vi "Test_Multiple_SubPanel_Single HSMO_External_Control.vi"() -> ()   [LabVIEW 2021]
uses:
  C:/Program Files (x86)/Hyper State Machine Framework/SSW_Hyper_State_Machine.lvlibp/State_Machine_Class/Main_State_Machine/Hyper_State_Machine.lvclass
  Commander/Commander.lvclass
  Image_Acquisition/Image_Acquisition.lvclass
  Motion_Control/Motion_Control.lvclass
  DIO/DIO.lvclass
  Data_Logging/Data_Logging.lvclass
  Common_State/Common_State.lvclass
  C:/Program Files (x86)/Hyper State Machine Framework/SSW_Hyper_State_Machine.lvlibp/State_Machine_Class/State_Machine_Module.llb/State Machine.ctl
  C:/Program Files (x86)/Hyper State Machine Framework/SSW_Hyper_State_Machine.lvlibp/State_Machine_Class/State_Machine_Module.llb/Lock_Unlock.ctl
  C:/Program Files (x86)/Hyper State Machine Framework/SSW_Hyper_State_Machine.lvlibp
panel:
  out "VI_Path[]":path[](array[path])
  in  "Panel List":i32(listbox)
  in  "Change SubPanel":bool
  out "HSMO[]":refnum<class "Hyper_State_Machine.lvclass">[](array[class])
  out "Lock Status":enum32{"Unlock", "Lock"}[](array[radio])
  in  "Lock State":bool
  in  "Change Mode":bool=TRUE
  in  "Panel Index":i32
  in  "Show Stop Button":bool
  in  "UnLoad_Panel":bool
  in  "Load_Panel":bool
  in  "Time Target (s)":dbl=30.0 format="%#_13g"
  in  "System_Delay(s)":dbl=0.01 format="%.0p"
  in  "State_Interval_Time(s)":dbl format="%.0p"
  in  "Stop":bool=TRUE
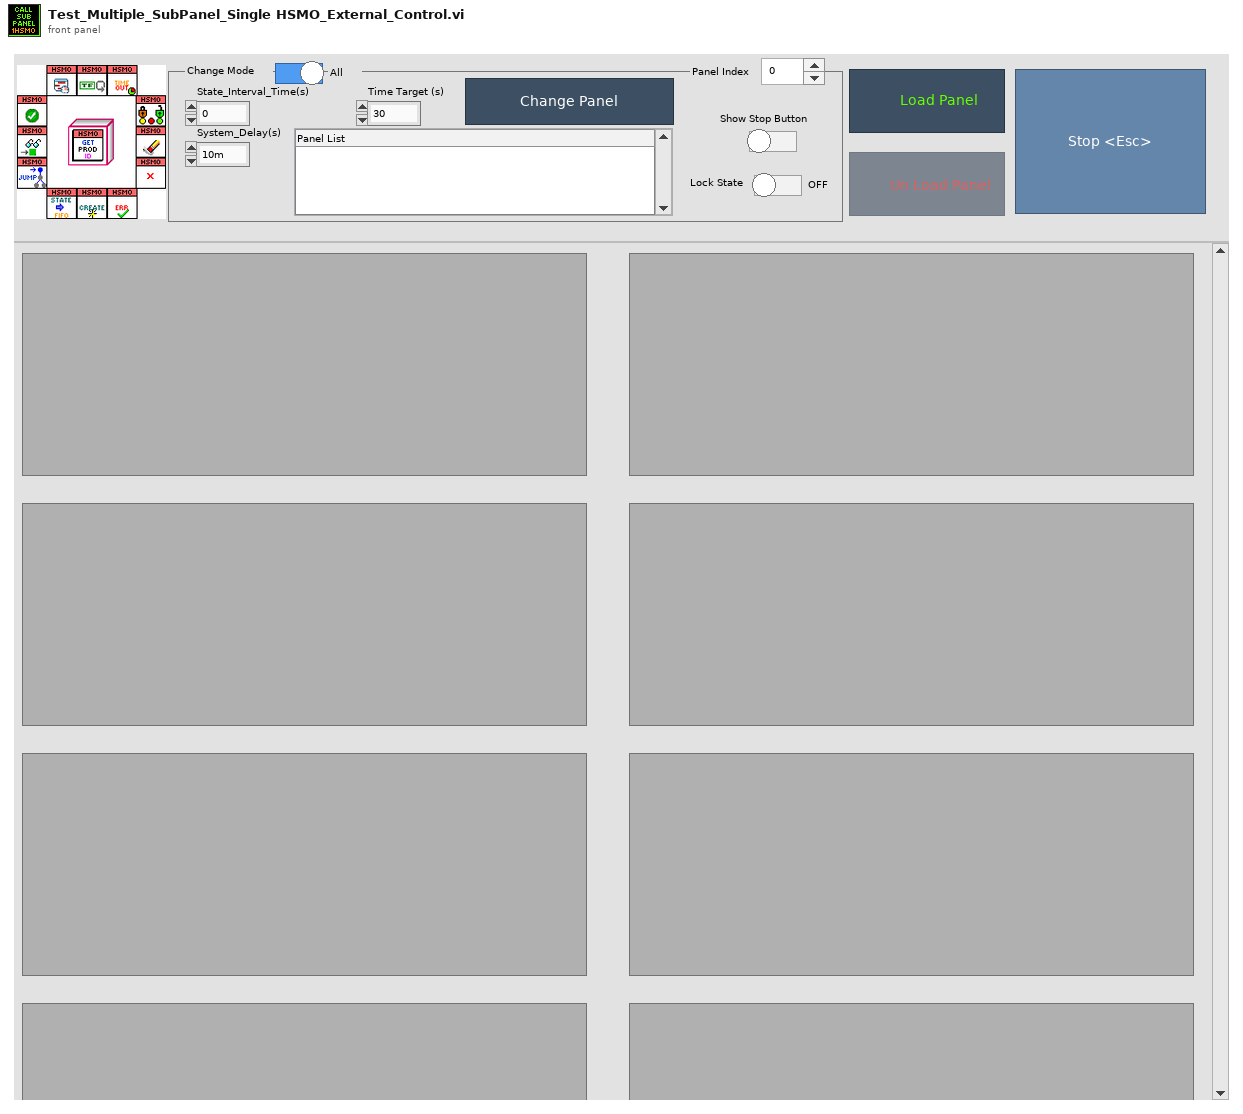
[diagram p1: front panel]
types:
  T1 = enum8{"Enabled", "Disabled", "Disabled and Grayed Out"}
  T2 = typedef "SSW_Hyper_State_Machine.lvlibp/State Machine.ctl" = cluster{"Command":string, "Data":variant}
  T3 = typedef "SSW_Hyper_State_Machine.lvlibp/Lock_Unlock.ctl" = cluster{"Action_Mode (Get)":enum16{"Set", "Get"}, "Action_Set (False)":bool, "State_In (Wait)":string}
  T4 = cluster{"data name":string, "drag data":variant}[]
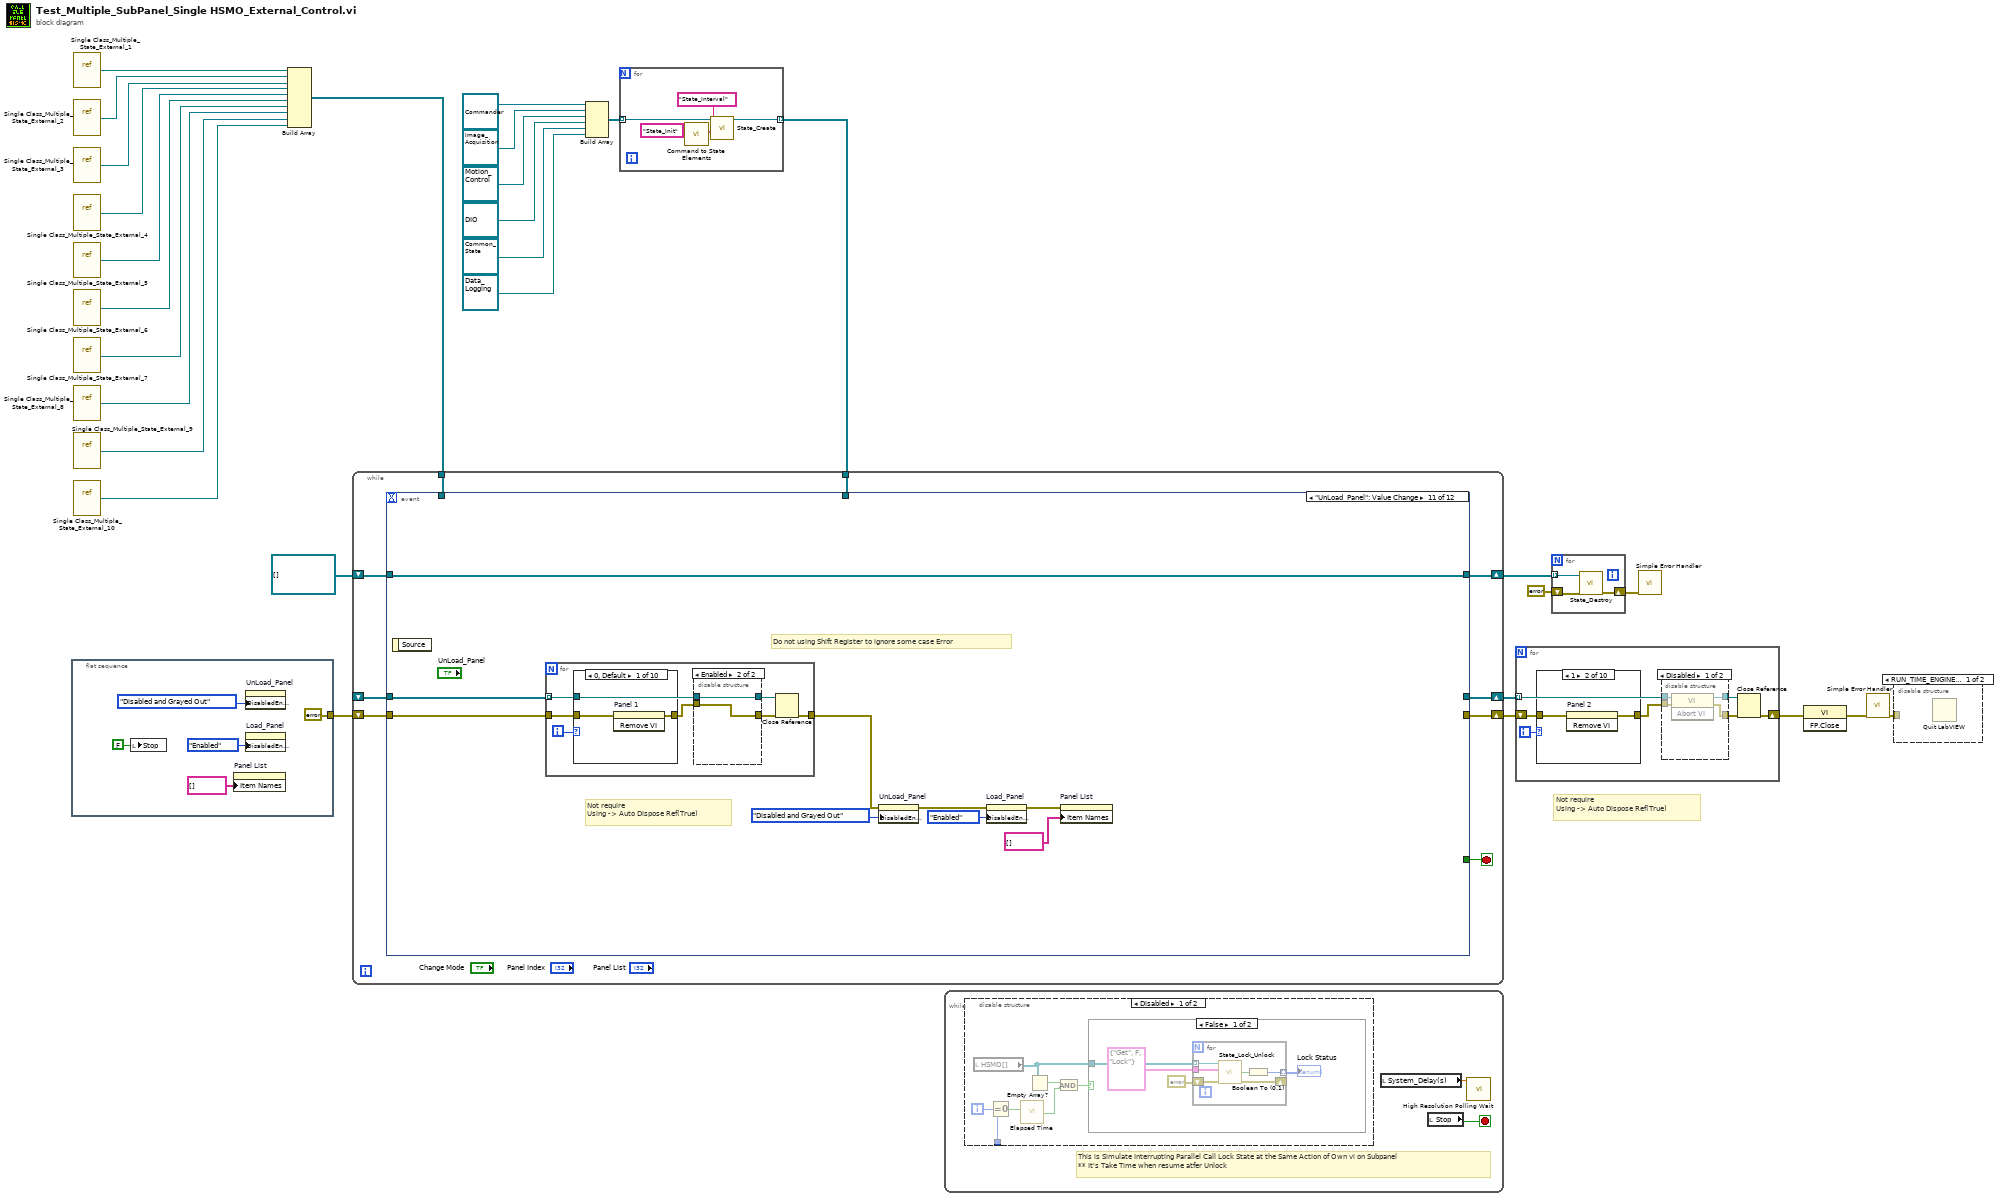
[diagram p0: block diagram]
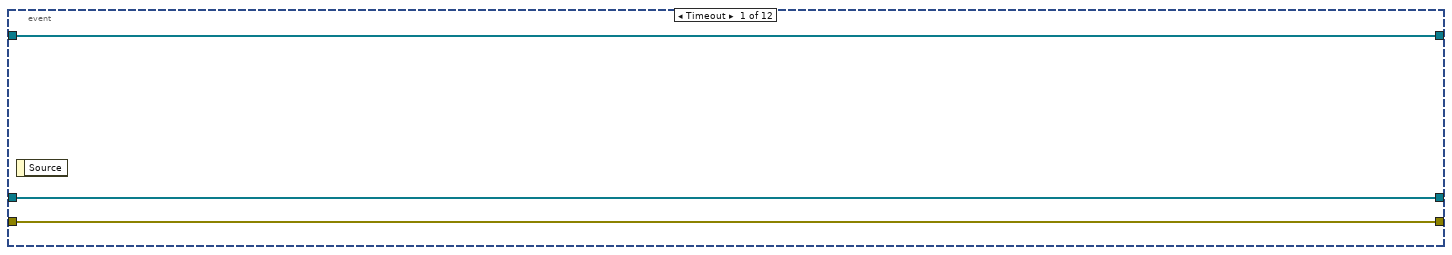
[diagram p5: hidden frame]
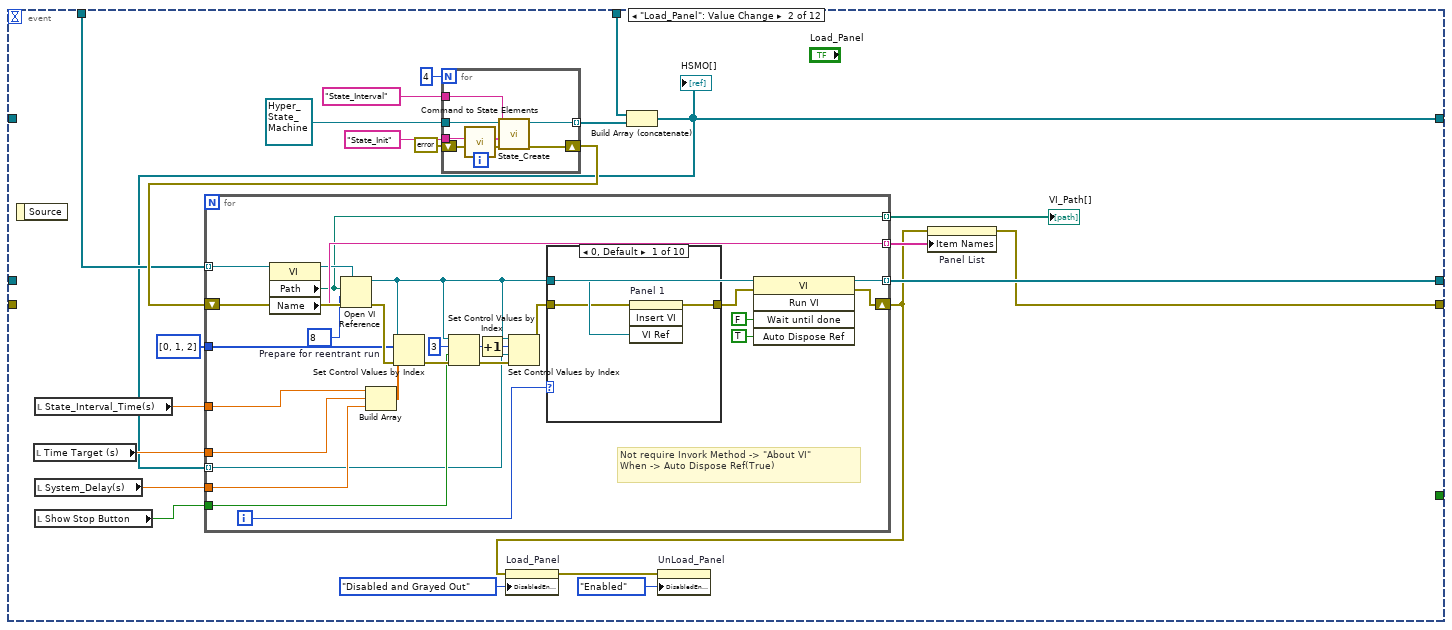
[diagram p6: hidden frame]
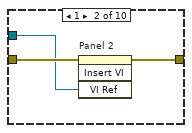
[diagram p7: hidden frame]
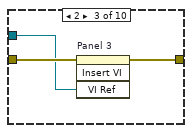
[diagram p8: hidden frame]
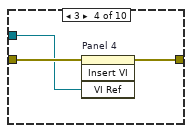
[diagram p9: hidden frame]
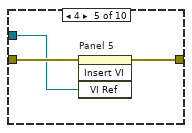
[diagram p10: hidden frame]
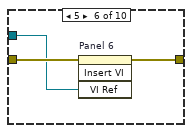
[diagram p11: hidden frame]
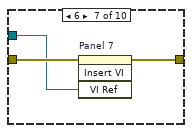
[diagram p12: hidden frame]
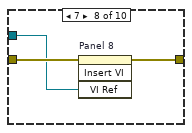
[diagram p13: hidden frame]
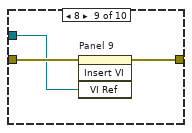
[diagram p14: hidden frame]
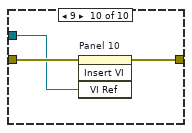
[diagram p15: hidden frame]
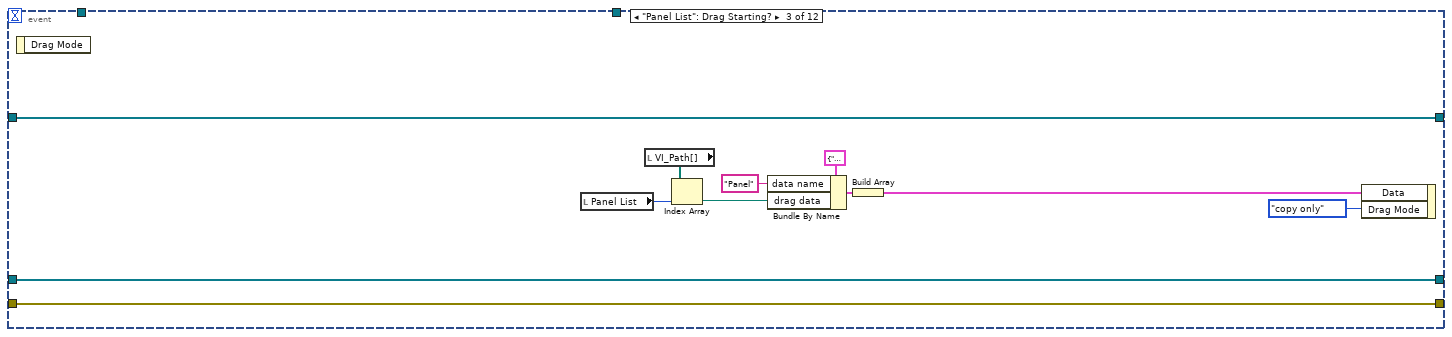
[diagram p16: hidden frame]
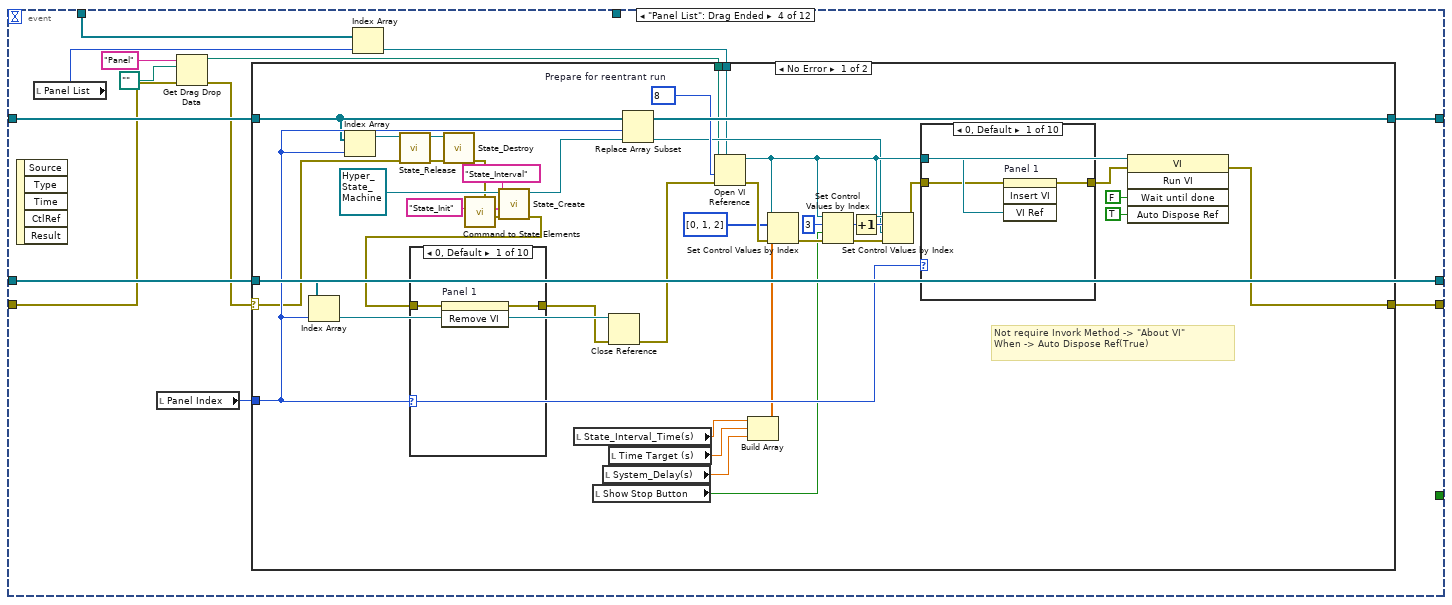
[diagram p17: hidden frame]
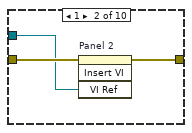
[diagram p18: hidden frame]
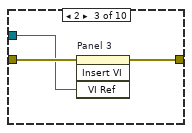
[diagram p19: hidden frame]
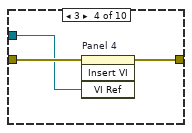
[diagram p20: hidden frame]
diagram:
  # "Not require\nUsing -> Auto Dispose Ref(True)"
  n1 = flat-sequence {
    tunnel: [errorcluster {"status"=FALSE, "code"=0, "source"=""} ("error out")] -> w27
    frame #0 {
      n2 = local write "Stop"(FALSE ("Stop")) -> ()
      n3 = property on="Panel List" class="LstBox (strict)"("Item Names"=string[] []) -> ()  [unwired: 2 in, 2 out]
      n4 = property on="UnLoad_Panel" class="Bool"("DisabledEnum"=T1."Disabled and Grayed Out" ("Disabled")) -> ()  [unwired: 2 in, 2 out]
      n5 = property on="Load_Panel" class="Bool"("DisabledEnum"=T1."Enabled" ("Disabled")) -> ()  [unwired: 2 in, 2 out]
    }
  }
  n6 = vi-ref "Single Class_Multiple_State_External_1.vi"() -> (w23:refnum<vi>)
  n7 = vi-ref "Single Class_Multiple_State_External_2.vi"() -> (w22:refnum<vi>)
  n8 = vi-ref "Single Class_Multiple_State_External_3.vi"() -> (w21:refnum<vi>)
  n9 = vi-ref "Single Class_Multiple_State_External_4.vi"() -> (w20:refnum<vi>)
  n10 = vi-ref "Single Class_Multiple_State_External_5.vi"() -> (w19:refnum<vi>)
  n11 = vi-ref "Single Class_Multiple_State_External_6.vi"() -> (w18:refnum<vi>)
  n12 = vi-ref "Single Class_Multiple_State_External_7.vi"() -> (w17:refnum<vi>)
  n13 = vi-ref "Single Class_Multiple_State_External_8.vi"() -> (w16:refnum<vi>)
  n14 = vi-ref "Single Class_Multiple_State_External_9.vi"() -> (w15:refnum<vi>)
  n15 = vi-ref "Single Class_Multiple_State_External_10.vi"() -> (w14:refnum<vi>)
  n16 = Build Array(w23, w22, w21, w20, w19, w18, w17, w16, w15, w14) -> (w13:refnum<vi>[])
  n17 = Build Array(refnum<class "Commander.lvclass"> refnum ("Commander.lvclass"), refnum<class "Image_Acquisition.lvclass"> refnum ("Image_Acquisition.lvclass"), refnum<class "Motion_Control.lvclass"> refnum ("Motion_Control.lvclass"), refnum<class "DIO.lvclass"> refnum ("DIO.lvclass"), refnum<class "Common_State.lvclass"> refnum ("Common_State.lvclass"), refnum<class "Data_Logging.lvclass"> refnum ("Data_Logging.lvclass")) -> (w7:refnum<class "Hyper_State_Machine.lvclass">[])
  n18 = for {
    tunnel: w7 -> [w36] mode=indexing
    tunnel: [w35] -> w1 mode=indexing
    n19 = call "Command to State Elements.vi"("Command"="State_Init") -> ("Command to State Elements"=w37:T2)  [unwired: 10 in]
    n20 = call-dynamic "State_Create.vi"("Init_State(Option)"=w37, "State_Interval_Name"="State_Interval" ("Core_Interval_Name(State_Interval)"), "State_Machine_Class in"=w36) -> ("State_Machine_Class out"=w35:refnum<class "Hyper_State_Machine.lvclass">)  [unwired: 6 in, 2 out]
  }
  n21 = while {
    shift-right: [w47] -> w29
    shift-left: _ -> [w46]
    shift-right: [w45] -> w28
    shift-left: w27 -> [w44]
    tunnel: w13 -> [w43]
    tunnel: w1 -> [w42]
    shift-right: [w41] -> w10
    shift-left: refnum<class "Hyper_State_Machine.lvclass">[] [] -> [w40]
    stop <- w48 stop-if-true
    n22 = event shown="[10] \"UnLoad_Panel\": Value Change" {
      selector: _ -> [_ _ _ _ _ _ _ _ _ _ _ _]
      dyn-events: _ -> [_ _ _ _ _ _ _ _ _ _ _ _]
      timeout: _ -> [_ _ _ _ _ _ _ _ _ _ _ _]
      tunnel: [_ _ _ _ _ _ _ _ _ _ _ w509] -> w48
      tunnel: [w51 w73 w142 w159 w257 w357 w380 w402 w425 w448 _ w510] -> w47
      tunnel: w46 -> [w51 _ w142 w159 w259 w357 w380 w402 w425 w448 w473 w510]
      tunnel: [w50 w53 w141 w158 w256 w356 w375 w401 w424 w447 _ w508] -> w45
      tunnel: w44 -> [w50 _ w141 w153 w260 w356 w375 w401 w424 w447 w469 w508]
      tunnel: w43 -> [_ w64 _ w152 _ _ _ _ _ _ _ _]
      tunnel: w42 -> [_ w57 _ _ _ _ _ _ _ _ _ _]
      tunnel: [w49 w56 w143 w157 w253 w352 w376 w396 w419 w442 w467 w507] -> w41
      tunnel: w40 -> [w49 _ w143 w160 w254 w352 w376 w396 w419 w442 w467 w507]
      event Timeout {
        n23 = event-data() -> ()  [unwired: 1 in, 1 out]
      }
      event "Load_Panel": Value Change {
        n24 = event-data() -> ()  [unwired: 1 in, 1 out]
        n25 = local read "Time Target (s)"() -> (w65:dbl)
        n26 = local read "State_Interval_Time(s)"() -> (w69:dbl)
        n27 = local read "System_Delay(s)"() -> (w67:dbl)
        n28 = local read "Show Stop Button"() -> (w66:bool)
        n29 = for {
          N: 4 -> [_]
          tunnel: refnum<class "Hyper_State_Machine.lvclass"> refnum ("SSW_Hyper_State_Machine.lvlibp:Hyper_State_Machine.lvclass") -> [w81]
          tunnel: "State_Init" ("Command") -> [w79]
          tunnel: "State_Interval" ("Core_Interval_Name(State_Interval)") -> [w78]
          shift-right: [w77] -> w68
          shift-left: errorcluster {"status"=FALSE, "code"=0, "source"=""} ("error out") -> [w76]
          tunnel: [w75] -> w58 mode=indexing
          n30 = call "Command to State Elements.vi"("Command"=w79) -> ("Command to State Elements"=w80:T2)  [unwired: 10 in]
          n31 = call-dynamic "State_Create.vi"("error in (no error)"=w76, "Init_State(Option)"=w80, "State_Interval_Name"=w78, "State_Machine_Class in"=w81) -> ("error out"=w77:errorcluster, "State_Machine_Class out"=w75:refnum<class "Hyper_State_Machine.lvclass">)  [unwired: 5 in, 1 out]
        }
        n32 = Build Array (concatenate)(w57, w58) -> (w56:refnum<class "Hyper_State_Machine.lvclass">[])
        "HSMO[]" <- w56
        n33 = for {
          shift-right: [w100] -> w54
          shift-left: w68 -> [w107]
          tunnel: w64 -> [w106] mode=indexing
          tunnel: [w102] -> w73 mode=indexing
          tunnel: w69 -> [w97]
          tunnel: w67 -> [w96]
          tunnel: w65 -> [w95]
          tunnel: i32[] [0, 1, 2] ("control indexes") -> [w94]
          tunnel: w66 -> [w93]
          tunnel: w56 -> [w86] mode=indexing
          tunnel: [w84] -> w55 mode=indexing
          tunnel: [w82] -> w52 mode=indexing
          i -> [w87]
          w90 = 3
          w85 = 8  # Prepare for reentrant run
          # "Not require Invork Method -> \"About VI\"\nWhen -> Auto Dispose Ref(True)"
          n34 = property class="VI"(reference=w106) -> (reference out=w83:refnum<vi>, "Path"=w82:path, "Name"=w84:string)  [unwired: 1 in, 1 out]
          n35 = Open VI Reference(type specifier VI Refnum (for type only)=w83, vi path=w82, options=w85, error in (no error)=w107) -> (vi reference=w88:refnum<vi>, error out=w105:errorcluster)  [unwired: 2 in]
          n36 = Build Array(w97, w95, w96) -> (w99:dbl[])
          n37 = Set Control Values by Index(0:w88, 1:w94, 2:w99, 3:w105) -> (11:w98:errorcluster)
          n38 = Set Control Values by Index(0:w88, 1:w90, 2:w93, 3:w98) -> (11:w92:errorcluster)
          n39 = Increment(x=w90) -> (x+1=w89:i32)
          n40 = Set Control Values by Index(0:w88, 1:w89, 2:w86, 3:w92) -> (11:w91:errorcluster)
          n41 = case shown="0, Default" w87 {
            tunnel: w91 -> [w108 w113 w116 w119 w122 w125 w128 w131 w134 w137]
            tunnel: w88 -> [w109 w112 w114 w117 w120 w123 w126 w129 w132 w135]
            tunnel: [w110 w111 w115 w118 w121 w124 w127 w130 w133 w136] -> w101
            frame 0, Default {
              n42 = invoke on="Panel 1" class="SubPnl" method="Insert VI"(error in=w108, "VI Ref"=w109) -> (error out=w110:errorcluster)  [unwired: 2 in, 3 out]
            }
            frame 1 {
              n43 = invoke on="Panel 2" class="SubPnl" method="Insert VI"(error in=w113, "VI Ref"=w112) -> (error out=w111:errorcluster)  [unwired: 2 in, 3 out]
            }
            frame 2 {
              n44 = invoke on="Panel 3" class="SubPnl" method="Insert VI"(error in=w116, "VI Ref"=w114) -> (error out=w115:errorcluster)  [unwired: 2 in, 3 out]
            }
            frame 3 {
              n45 = invoke on="Panel 4" class="SubPnl" method="Insert VI"(error in=w119, "VI Ref"=w117) -> (error out=w118:errorcluster)  [unwired: 2 in, 3 out]
            }
            frame 4 {
              n46 = invoke on="Panel 5" class="SubPnl" method="Insert VI"(error in=w122, "VI Ref"=w120) -> (error out=w121:errorcluster)  [unwired: 2 in, 3 out]
            }
            frame 5 {
              n47 = invoke on="Panel 6" class="SubPnl" method="Insert VI"(error in=w125, "VI Ref"=w123) -> (error out=w124:errorcluster)  [unwired: 2 in, 3 out]
            }
            frame 6 {
              n48 = invoke on="Panel 7" class="SubPnl" method="Insert VI"(error in=w128, "VI Ref"=w126) -> (error out=w127:errorcluster)  [unwired: 2 in, 3 out]
            }
            frame 7 {
              n49 = invoke on="Panel 8" class="SubPnl" method="Insert VI"(error in=w131, "VI Ref"=w129) -> (error out=w130:errorcluster)  [unwired: 2 in, 3 out]
            }
            frame 8 {
              n50 = invoke on="Panel 9" class="SubPnl" method="Insert VI"(error in=w134, "VI Ref"=w132) -> (error out=w133:errorcluster)  [unwired: 2 in, 3 out]
            }
            frame 9 {
              n51 = invoke on="Panel 10" class="SubPnl" method="Insert VI"(error in=w137, "VI Ref"=w135) -> (error out=w136:errorcluster)  [unwired: 2 in, 3 out]
            }
          }
          n52 = invoke class="VI" method="Run VI"(reference=w88, error in=w101, "Wait until done"=FALSE ("Wait Until Done"), "Auto Dispose Ref"=TRUE ("Auto Dispose Reference")) -> (reference out=w102:refnum<vi>, error out=w100:errorcluster)  [unwired: 1 in, 3 out]
        }
        "VI_Path[]" <- w52
        n53 = property on="Load_Panel" class="Bool"(error in=w54, "DisabledEnum"=T1."Disabled and Grayed Out" ("Disabled")) -> (error out=w70:errorcluster)  [unwired: 1 in, 1 out]
        n54 = property on="UnLoad_Panel" class="Bool"(error in=w70, "DisabledEnum"=T1."Enabled" ("Disabled")) -> ()  [unwired: 1 in, 2 out]
        n55 = property on="Panel List" class="LstBox (strict)"(error in=w54, "Item Names"=w55) -> (error out=w53:errorcluster)  [unwired: 1 in, 1 out]
      }
      event "Panel List": Drag Starting? {
        n56 = event-data() -> ()  [unwired: 1 in, 1 out]
        n57 = local read "Panel List"() -> (w139:i32)
        n58 = local read "VI_Path[]"() -> (w140:path[])
        n59 = Index Array(array=w140, index=w139) -> (element=w138:path)
        n60 = Bundle By Name(cluster=cluster{"data name":string, "drag data":variant} {"data name"="", "drag data"=variant}, "data name"="Panel", "drag data"=w138) -> (w145:cluster{"data name":string, "drag data":variant})
        n61 = Build Array(w145) -> (w144:T4)
        n62 = event-data("Data"=w144, "Drag Mode"=enum32{"copy or move", "copy only", "move only"}."copy only") -> ()  [unwired: 1 in, 1 out]
      }
      event "Panel List": Drag Ended {
        n63 = event-data() -> ()  [unwired: 1 in, 5 out]
        n64 = local read "Panel List"() -> (w151:i32)
        n65 = local read "Panel Index"() -> (w161:i32)
        n66 = Get Drag Drop Data(6:w153, 8:path "" ("element"), 9:"Panel" ("data name")) -> (0:w149:errorcluster, 3:w154:path)
        n67 = Index Array(array=w152, index=w151) -> (element=w150:refnum<vi>)
        n68 = case shown="No Error" w149 {
          selector: w149 -> [w162 w250]
          tunnel: w161 -> [w199 _]
          tunnel: w160 -> [w198 w251]
          tunnel: w159 -> [w197 _]
          tunnel: [w196 w250] -> w158
          tunnel: [w195 w251] -> w157
          tunnel: w154 -> [w164 _]
          tunnel: w150 -> [w163 _]
          frame No Error {
            w182 = 3
            w178 = 8  # Prepare for reentrant run
            # "Not require Invork Method -> \"About VI\"\nWhen -> Auto Dispose Ref(True)"
            n69 = Index Array(array=w197, index=w199) -> (element=w167:refnum<vi>)
            n70 = Index Array(array=w198, index=w199) -> (element=w173:refnum<class "Hyper_State_Machine.lvclass">)
            n71 = call-dynamic "State_Release.vi"("error in (no error)"=w162, "State_Machine_Class in"=w173) -> ("error out"=w172:errorcluster, "State_Machine_Class out"=w171:refnum<class "Hyper_State_Machine.lvclass">)  [unwired: 8 in]
            n72 = call-dynamic "State_Destroy.vi"("error in (no error)"=w172, "State_Machine_Class in"=w171) -> ("error out"=w170:errorcluster)  [unwired: 9 in]
            n73 = call "Command to State Elements.vi"("Command"="State_Init") -> ("Command to State Elements"=w177:T2)  [unwired: 10 in]
            n74 = call-dynamic "State_Create.vi"("error in (no error)"=w170, "Init_State(Option)"=w177, "State_Interval_Name"="State_Interval" ("Core_Interval_Name(State_Interval)"), "State_Machine_Class in"=refnum<class "Hyper_State_Machine.lvclass"> refnum ("State_Machine_Class out")) -> ("error out"=w168:errorcluster, "State_Machine_Class out"=w169:refnum<class "Hyper_State_Machine.lvclass">)  [unwired: 5 in, 1 out]
            n75 = case shown="0, Default" w199 {
              tunnel: w168 -> [w230 w233 w235 w237 w239 w241 w243 w245 w247 w249]
              tunnel: [w231 w232 w234 w236 w238 w240 w242 w244 w246 w248] -> w166
              frame 0, Default {
                n76 = invoke on="Panel 1" class="SubPnl" method="Remove VI"(error in=w230) -> (error out=w231:errorcluster)  [unwired: 2 in, 2 out]
              }
              frame 1 {
                n77 = invoke on="Panel 2" class="SubPnl" method="Remove VI"(error in=w233) -> (error out=w232:errorcluster)  [unwired: 2 in, 2 out]
              }
              frame 2 {
                n78 = invoke on="Panel 3" class="SubPnl" method="Remove VI"(error in=w235) -> (error out=w234:errorcluster)  [unwired: 2 in, 2 out]
              }
              frame 3 {
                n79 = invoke on="Panel 4" class="SubPnl" method="Remove VI"(error in=w237) -> (error out=w236:errorcluster)  [unwired: 2 in, 2 out]
              }
              frame 4 {
                n80 = invoke on="Panel 5" class="SubPnl" method="Remove VI"(error in=w239) -> (error out=w238:errorcluster)  [unwired: 2 in, 2 out]
              }
              frame 5 {
                n81 = invoke on="Panel 6" class="SubPnl" method="Remove VI"(error in=w241) -> (error out=w240:errorcluster)  [unwired: 2 in, 2 out]
              }
              frame 6 {
                n82 = invoke on="Panel 7" class="SubPnl" method="Remove VI"(error in=w243) -> (error out=w242:errorcluster)  [unwired: 2 in, 2 out]
              }
              frame 7 {
                n83 = invoke on="Panel 8" class="SubPnl" method="Remove VI"(error in=w245) -> (error out=w244:errorcluster)  [unwired: 2 in, 2 out]
              }
              frame 8 {
                n84 = invoke on="Panel 9" class="SubPnl" method="Remove VI"(error in=w247) -> (error out=w246:errorcluster)  [unwired: 2 in, 2 out]
              }
              frame 9 {
                n85 = invoke on="Panel 10" class="SubPnl" method="Remove VI"(error in=w249) -> (error out=w248:errorcluster)  [unwired: 2 in, 2 out]
              }
            }
            n86 = local read "State_Interval_Time(s)"() -> (w186:dbl)
            n87 = local read "Show Stop Button"() -> (w184:bool)
            n88 = local read "System_Delay(s)"() -> (w185:dbl)
            n89 = Close Reference(reference=w167, error in (no error)=w166) -> (error out=w165:errorcluster)
            n90 = local read "Time Target (s)"() -> (w183:dbl)
            n91 = Replace Array Subset(array=w198, new element=w169, index=w199) -> (w195:refnum<class "Hyper_State_Machine.lvclass">[])
            n92 = Open VI Reference(type specifier VI Refnum (for type only)=w163, vi path=w164, options=w178, error in (no error)=w165) -> (vi reference=w194:refnum<vi>, error out=w187:errorcluster)  [unwired: 2 in]
            n93 = Build Array(w186, w183, w185) -> (w189:dbl[])
            n94 = Set Control Values by Index(0:w194, 1:i32[] [0, 1, 2] ("control indexes"), 2:w189, 3:w187) -> (11:w190:errorcluster)
            n95 = Set Control Values by Index(0:w194, 1:w182, 2:w184, 3:w190) -> (11:w191:errorcluster)
            n96 = Increment(x=w182) -> (x+1=w193:i32)
            n97 = Set Control Values by Index(0:w194, 1:w193, 2:w169, 3:w191) -> (11:w192:errorcluster)
            n98 = case shown="0, Default" w199 {
              tunnel: w192 -> [w200 w205 w208 w211 w214 w217 w220 w223 w226 w229]
              tunnel: w194 -> [w201 w204 w206 w209 w212 w215 w218 w221 w224 w227]
              tunnel: [w202 w203 w207 w210 w213 w216 w219 w222 w225 w228] -> w188
              frame 0, Default {
                n99 = invoke on="Panel 1" class="SubPnl" method="Insert VI"(error in=w200, "VI Ref"=w201) -> (error out=w202:errorcluster)  [unwired: 2 in, 3 out]
              }
              frame 1 {
                n100 = invoke on="Panel 2" class="SubPnl" method="Insert VI"(error in=w205, "VI Ref"=w204) -> (error out=w203:errorcluster)  [unwired: 2 in, 3 out]
              }
              frame 2 {
                n101 = invoke on="Panel 3" class="SubPnl" method="Insert VI"(error in=w208, "VI Ref"=w206) -> (error out=w207:errorcluster)  [unwired: 2 in, 3 out]
              }
              frame 3 {
                n102 = invoke on="Panel 4" class="SubPnl" method="Insert VI"(error in=w211, "VI Ref"=w209) -> (error out=w210:errorcluster)  [unwired: 2 in, 3 out]
              }
              frame 4 {
                n103 = invoke on="Panel 5" class="SubPnl" method="Insert VI"(error in=w214, "VI Ref"=w212) -> (error out=w213:errorcluster)  [unwired: 2 in, 3 out]
              }
              frame 5 {
                n104 = invoke on="Panel 6" class="SubPnl" method="Insert VI"(error in=w217, "VI Ref"=w215) -> (error out=w216:errorcluster)  [unwired: 2 in, 3 out]
              }
              frame 6 {
                n105 = invoke on="Panel 7" class="SubPnl" method="Insert VI"(error in=w220, "VI Ref"=w218) -> (error out=w219:errorcluster)  [unwired: 2 in, 3 out]
              }
              frame 7 {
                n106 = invoke on="Panel 8" class="SubPnl" method="Insert VI"(error in=w223, "VI Ref"=w221) -> (error out=w222:errorcluster)  [unwired: 2 in, 3 out]
              }
              frame 8 {
                n107 = invoke on="Panel 9" class="SubPnl" method="Insert VI"(error in=w226, "VI Ref"=w224) -> (error out=w225:errorcluster)  [unwired: 2 in, 3 out]
              }
              frame 9 {
                n108 = invoke on="Panel 10" class="SubPnl" method="Insert VI"(error in=w229, "VI Ref"=w227) -> (error out=w228:errorcluster)  [unwired: 2 in, 3 out]
              }
            }
            n109 = invoke class="VI" method="Run VI"(reference=w194, error in=w188, "Wait until done"=FALSE ("Wait Until Done"), "Auto Dispose Ref"=TRUE ("Auto Dispose Reference")) -> (error out=w196:errorcluster)  [unwired: 1 in, 4 out]
          }
          frame Error {
          }
        }
      }
      event "Change SubPanel": Value Change {
        n110 = event-data() -> ()  [unwired: 1 in, 1 out]
        n111 = local read "Panel Index"() -> (w261:i32)
        n112 = call "File Dialog"("prompt"="Select vi to Loading . . .") -> ("selected path"=w255:path, "cancelled"=w258:bool)  [unwired: 11 in, 2 out]
        n113 = case shown="False" w258 {
          tunnel: w261 -> [w266 _]
          tunnel: w260 -> [w272 w350]
          tunnel: [w267 w351] -> w257
          tunnel: w259 -> [w267 w351]
          tunnel: [w280 w350] -> w256
          tunnel: w255 -> [w281 _]
          tunnel: w254 -> [w270 w349]
          tunnel: [w269 w349] -> w253
          frame False {
            w286 = 3
            w282 = 8  # Prepare for reentrant run
            # "Not require Invork Method -> \"About VI\"\nWhen -> Auto Dispose Ref(True)"
            n114 = Index Array(array=w267, index=w266) -> (element=w264:refnum<vi>)
            n115 = Index Array(array=w270, index=w266) -> (element=w275:refnum<class "Hyper_State_Machine.lvclass">)
            n116 = call-dynamic "State_Release.vi"("error in (no error)"=w272, "State_Machine_Class in"=w275) -> ("error out"=w274:errorcluster, "State_Machine_Class out"=w273:refnum<class "Hyper_State_Machine.lvclass">)  [unwired: 8 in]
            n117 = call-dynamic "State_Destroy.vi"("error in (no error)"=w274, "State_Machine_Class in"=w273) -> ("error out"=w271:errorcluster)  [unwired: 9 in]
            n118 = call "Command to State Elements.vi"("Command"="State_Init") -> ("Command to State Elements"=w279:T2)  [unwired: 10 in]
            n119 = call-dynamic "State_Create.vi"("error in (no error)"=w271, "Init_State(Option)"=w279, "State_Interval_Name"="State_Interval" ("Core_Interval_Name(State_Interval)"), "State_Machine_Class in"=refnum<class "Hyper_State_Machine.lvclass"> refnum ("State_Machine_Class out")) -> ("error out"=w265:errorcluster, "State_Machine_Class out"=w268:refnum<class "Hyper_State_Machine.lvclass">)  [unwired: 5 in, 1 out]
            n120 = case shown="0, Default" w266 {
              tunnel: w265 -> [w329 w332 w334 w336 w338 w340 w342 w344 w346 w348]
              tunnel: [w330 w331 w333 w335 w337 w339 w341 w343 w345 w347] -> w263
              frame 0, Default {
                n121 = invoke on="Panel 1" class="SubPnl" method="Remove VI"(error in=w329) -> (error out=w330:errorcluster)  [unwired: 2 in, 2 out]
              }
              frame 1 {
                n122 = invoke on="Panel 2" class="SubPnl" method="Remove VI"(error in=w332) -> (error out=w331:errorcluster)  [unwired: 2 in, 2 out]
              }
              frame 2 {
                n123 = invoke on="Panel 3" class="SubPnl" method="Remove VI"(error in=w334) -> (error out=w333:errorcluster)  [unwired: 2 in, 2 out]
              }
              frame 3 {
                n124 = invoke on="Panel 4" class="SubPnl" method="Remove VI"(error in=w336) -> (error out=w335:errorcluster)  [unwired: 2 in, 2 out]
              }
              frame 4 {
                n125 = invoke on="Panel 5" class="SubPnl" method="Remove VI"(error in=w338) -> (error out=w337:errorcluster)  [unwired: 2 in, 2 out]
              }
              frame 5 {
                n126 = invoke on="Panel 6" class="SubPnl" method="Remove VI"(error in=w340) -> (error out=w339:errorcluster)  [unwired: 2 in, 2 out]
              }
              frame 6 {
                n127 = invoke on="Panel 7" class="SubPnl" method="Remove VI"(error in=w342) -> (error out=w341:errorcluster)  [unwired: 2 in, 2 out]
              }
              frame 7 {
                n128 = invoke on="Panel 8" class="SubPnl" method="Remove VI"(error in=w344) -> (error out=w343:errorcluster)  [unwired: 2 in, 2 out]
              }
              frame 8 {
                n129 = invoke on="Panel 9" class="SubPnl" method="Remove VI"(error in=w346) -> (error out=w345:errorcluster)  [unwired: 2 in, 2 out]
              }
              frame 9 {
                n130 = invoke on="Panel 10" class="SubPnl" method="Remove VI"(error in=w348) -> (error out=w347:errorcluster)  [unwired: 2 in, 2 out]
              }
            }
            n131 = local read "State_Interval_Time(s)"() -> (w290:dbl)
            n132 = local read "Show Stop Button"() -> (w288:bool)
            n133 = local read "System_Delay(s)"() -> (w289:dbl)
            n134 = Close Reference(reference=w264, error in (no error)=w263) -> (error out=w262:errorcluster)
            n135 = local read "Time Target (s)"() -> (w287:dbl)
            n136 = Replace Array Subset(array=w270, new element=w268, index=w266) -> (w269:refnum<class "Hyper_State_Machine.lvclass">[])
            n137 = Open VI Reference(vi path=w281, options=w282, error in (no error)=w262) -> (vi reference=w298:refnum<vi>, error out=w291:errorcluster)  [unwired: 3 in]
            n138 = Build Array(w290, w287, w289) -> (w293:dbl[])
            n139 = Set Control Values by Index(0:w298, 1:i32[] [0, 1, 2] ("control indexes"), 2:w293, 3:w291) -> (11:w294:errorcluster)
            n140 = Set Control Values by Index(0:w298, 1:w286, 2:w288, 3:w294) -> (11:w295:errorcluster)
            n141 = Increment(x=w286) -> (x+1=w297:i32)
            n142 = Set Control Values by Index(0:w298, 1:w297, 2:w268, 3:w295) -> (11:w296:errorcluster)
            n143 = case shown="0, Default" w266 {
              tunnel: w296 -> [w299 w304 w307 w310 w313 w316 w319 w322 w325 w328]
              tunnel: w298 -> [w300 w303 w305 w308 w311 w314 w317 w320 w323 w326]
              tunnel: [w301 w302 w306 w309 w312 w315 w318 w321 w324 w327] -> w292
              frame 0, Default {
                n144 = invoke on="Panel 1" class="SubPnl" method="Insert VI"(error in=w299, "VI Ref"=w300) -> (error out=w301:errorcluster)  [unwired: 2 in, 3 out]
              }
              frame 1 {
                n145 = invoke on="Panel 2" class="SubPnl" method="Insert VI"(error in=w304, "VI Ref"=w303) -> (error out=w302:errorcluster)  [unwired: 2 in, 3 out]
              }
              frame 2 {
                n146 = invoke on="Panel 3" class="SubPnl" method="Insert VI"(error in=w307, "VI Ref"=w305) -> (error out=w306:errorcluster)  [unwired: 2 in, 3 out]
              }
              frame 3 {
                n147 = invoke on="Panel 4" class="SubPnl" method="Insert VI"(error in=w310, "VI Ref"=w308) -> (error out=w309:errorcluster)  [unwired: 2 in, 3 out]
              }
              frame 4 {
                n148 = invoke on="Panel 5" class="SubPnl" method="Insert VI"(error in=w313, "VI Ref"=w311) -> (error out=w312:errorcluster)  [unwired: 2 in, 3 out]
              }
              frame 5 {
                n149 = invoke on="Panel 6" class="SubPnl" method="Insert VI"(error in=w316, "VI Ref"=w314) -> (error out=w315:errorcluster)  [unwired: 2 in, 3 out]
              }
              frame 6 {
                n150 = invoke on="Panel 7" class="SubPnl" method="Insert VI"(error in=w319, "VI Ref"=w317) -> (error out=w318:errorcluster)  [unwired: 2 in, 3 out]
              }
              frame 7 {
                n151 = invoke on="Panel 8" class="SubPnl" method="Insert VI"(error in=w322, "VI Ref"=w320) -> (error out=w321:errorcluster)  [unwired: 2 in, 3 out]
              }
              frame 8 {
                n152 = invoke on="Panel 9" class="SubPnl" method="Insert VI"(error in=w325, "VI Ref"=w323) -> (error out=w324:errorcluster)  [unwired: 2 in, 3 out]
              }
              frame 9 {
                n153 = invoke on="Panel 10" class="SubPnl" method="Insert VI"(error in=w328, "VI Ref"=w326) -> (error out=w327:errorcluster)  [unwired: 2 in, 3 out]
              }
            }
            n154 = invoke class="VI" method="Run VI"(reference=w298, error in=w292, "Wait until done"=FALSE ("Wait Until Done"), "Auto Dispose Ref"=TRUE ("Auto Dispose Reference")) -> (error out=w280:errorcluster)  [unwired: 1 in, 4 out]
          }
          frame True {
          }
        }
      }
      event "State_Interval_Time(s)": Value Change {
        # "Change Only First State Member for Faster Access Time and Donot Duplicate the Same Target"
        n155 = event-data() -> ("NewVal"=w358:dbl)  [unwired: 1 in]
        n156 = local read "Change Mode"() -> (w354:bool)
        n157 = local read "Panel Index"() -> (w353:i32)
        n158 = Index Array(array=w352, index=w353) -> (element=w355:refnum<class "Hyper_State_Machine.lvclass">)
        n159 = case shown="True" w354 {
          tunnel: w358 -> [w362 w374]
          tunnel: w352 -> [w359 _]
          tunnel: w355 -> [_ w373]
          frame True {
            n160 = for {
              tunnel: w359 -> [w365] mode=indexing
              tunnel: w362 -> [w368]
              shift-right: [w367] -> _
              shift-left: errorcluster {"status"=FALSE, "code"=0, "source"=""} ("error out") -> [w364]
              tunnel: T2 {"Command"="Change_Interval_Value", "Data"=variant} ("State Machine") -> [w366]
              n161 = Bundle By Name(cluster=w366, "Data"=w368) -> (w369:T2)
              n162 = call-dynamic "State_LIFO.vi"("error in (no error)"=w364, "State_Interval(Enable)"=FALSE, "State Machine"=w369, "State_Machine_Class in"=w365) -> ("error out"=w367:errorcluster)  [unwired: 6 in, 1 out]
            }
          }
          frame False {
            n163 = Bundle By Name(cluster=T2 {"Command"="Change_Interval_Value", "Data"=variant} ("State Machine"), "Data"=w374) -> (w371:T2)
            n164 = call-dynamic "State_LIFO.vi"("State_Interval(Enable)"=FALSE, "State Machine"=w371, "State_Machine_Class in"=w373) -> ()  [unwired: 7 in, 2 out]
          }
        }
      }
      event "Lock State": Value Change {
        # "Change Only First State Member for Faster Access Time and Donot Duplicate the Same Target"
        n165 = event-data() -> ("NewVal"=w381:bool)  [unwired: 1 in]
        n166 = local read "Change Mode"() -> (w378:bool)
        n167 = local read "Panel Index"() -> (w377:i32)
        n168 = Index Array(array=w376, index=w377) -> (element=w379:refnum<class "Hyper_State_Machine.lvclass">)
        n169 = case shown="False" w378 {
          tunnel: w381 -> [w384 w395]
          tunnel: w376 -> [w386 _]
          tunnel: w379 -> [_ w393]
          tunnel: w375 -> [w382 w391]
          frame True {
            n170 = Bundle By Name(cluster=T3 {"Action_Mode (Get)"=enum."Set", "Action_Set (False)"=TRUE, "State_In (Wait)"="Lock"} ("Parameter"), "Action_Set (False)"=w384) -> (w383:T3)
            n171 = for {
              tunnel: w386 -> [w390] mode=indexing
              shift-right: [w387] -> _
              shift-left: w382 -> [w388]
              tunnel: w383 -> [w389]
              n172 = call-dynamic "State_Lock_Unlock.vi"("error in (no error)"=w388, "Parameter"=w389, "State_Machine_Class in"=w390) -> ("error out"=w387:errorcluster)  [unwired: 6 in, 2 out]
            }
          }
          frame False {
            n173 = Bundle By Name(cluster=T3 {"Action_Mode (Get)"=enum."Set", "Action_Set (False)"=TRUE, "State_In (Wait)"="Lock"} ("Parameter"), "Action_Set (False)"=w395) -> (w392:T3)
            n174 = call-dynamic "State_Lock_Unlock.vi"("error in (no error)"=w391, "Parameter"=w392, "State_Machine_Class in"=w393) -> ()  [unwired: 6 in, 3 out]
          }
        }
      }
      event "System_Delay(s)": Value Change {
        # "Change Only First State Member for Faster Access Time and Donot Duplicate the Same Target"
        n175 = event-data() -> ("NewVal"=w399:dbl)  [unwired: 1 in]
        n176 = local read "Change Mode"() -> (w398:bool)
        n177 = local read "Panel Index"() -> (w397:i32)
        n178 = Index Array(array=w396, index=w397) -> (element=w400:refnum<class "Hyper_State_Machine.lvclass">)
        n179 = case shown="False" w398 {
          tunnel: w399 -> [w406 w418]
          tunnel: w396 -> [w403 _]
          tunnel: w400 -> [_ w417]
          frame True {
            n180 = for {
              tunnel: w403 -> [w409] mode=indexing
              tunnel: w406 -> [w412]
              shift-right: [w411] -> _
              shift-left: errorcluster {"status"=FALSE, "code"=0, "source"=""} ("error out") -> [w408]
              tunnel: T2 {"Command"="Change_System_Delay", "Data"=variant} ("State Machine") -> [w410]
              n181 = Bundle By Name(cluster=w410, "Data"=w412) -> (w413:T2)
              n182 = call-dynamic "State_LIFO.vi"("error in (no error)"=w408, "State_Interval(Enable)"=FALSE, "State Machine"=w413, "State_Machine_Class in"=w409) -> ("error out"=w411:errorcluster)  [unwired: 6 in, 1 out]
            }
          }
          frame False {
            n183 = Bundle By Name(cluster=T2 {"Command"="Change_System_Delay", "Data"=variant} ("State Machine"), "Data"=w418) -> (w415:T2)
            n184 = call-dynamic "State_LIFO.vi"("State_Interval(Enable)"=FALSE, "State Machine"=w415, "State_Machine_Class in"=w417) -> ()  [unwired: 7 in, 2 out]
          }
        }
      }
      event "Time Target (s)": Value Change {
        # "Change Only First State Member for Faster Access Time and Donot Duplicate the Same Target"
        n185 = event-data() -> ("NewVal"=w422:dbl)  [unwired: 1 in]
        n186 = local read "Change Mode"() -> (w421:bool)
        n187 = local read "Panel Index"() -> (w420:i32)
        n188 = Index Array(array=w419, index=w420) -> (element=w423:refnum<class "Hyper_State_Machine.lvclass">)
        n189 = case shown="True" w421 {
          tunnel: w422 -> [w429 w441]
          tunnel: w419 -> [w426 _]
          tunnel: w423 -> [_ w440]
          frame True {
            n190 = for {
              tunnel: w426 -> [w432] mode=indexing
              tunnel: w429 -> [w435]
              shift-right: [w434] -> _
              shift-left: errorcluster {"status"=FALSE, "code"=0, "source"=""} ("error out") -> [w431]
              tunnel: T2 {"Command"="Change_Time_Target", "Data"=variant} ("State Machine") -> [w433]
              n191 = Bundle By Name(cluster=w433, "Data"=w435) -> (w436:T2)
              n192 = call-dynamic "State_LIFO.vi"("error in (no error)"=w431, "State_Interval(Enable)"=FALSE, "State Machine"=w436, "State_Machine_Class in"=w432) -> ("error out"=w434:errorcluster)  [unwired: 6 in, 1 out]
            }
          }
          frame False {
            n193 = Bundle By Name(cluster=T2 {"Command"="Change_Time_Target", "Data"=variant} ("State Machine"), "Data"=w441) -> (w438:T2)
            n194 = call-dynamic "State_LIFO.vi"("State_Interval(Enable)"=FALSE, "State Machine"=w438, "State_Machine_Class in"=w440) -> ()  [unwired: 7 in, 2 out]
          }
        }
      }
      event "Show Stop Button": Value Change {
        # "Change Only First State Member for Faster Access Time and Donot Duplicate the Same Target"
        n195 = event-data() -> ("NewVal"=w445:bool)  [unwired: 1 in]
        n196 = local read "Change Mode"() -> (w443:bool)
        n197 = local read "Panel Index"() -> (w444:i32)
        n198 = Index Array(array=w442, index=w444) -> (element=w446:refnum<class "Hyper_State_Machine.lvclass">)
        n199 = case shown="True" w443 {
          tunnel: w445 -> [w452 w464]
          tunnel: w446 -> [_ w460]
          tunnel: w442 -> [w449 _]
          frame True {
            n200 = for {
              tunnel: w452 -> [w459]
              tunnel: T2 {"Command"="Show_Stop_Button", "Data"=variant} ("State Machine") -> [w456]
              shift-right: [w457] -> _
              shift-left: errorcluster {"status"=FALSE, "code"=0, "source"=""} ("error out") -> [w458]
              tunnel: w449 -> [w453] mode=indexing
              n201 = Bundle By Name(cluster=w456, "Data"=w459) -> (w455:T2)
              n202 = call-dynamic "State_LIFO.vi"("error in (no error)"=w458, "State_Interval(Enable)"=FALSE, "State Machine"=w455, "State_Machine_Class in"=w453) -> ("error out"=w457:errorcluster)  [unwired: 6 in, 1 out]
            }
          }
          frame False {
            n203 = Bundle By Name(cluster=T2 {"Command"="Show_Stop_Button", "Data"=variant} ("State Machine"), "Data"=w464) -> (w462:T2)
            n204 = call-dynamic "State_LIFO.vi"("State_Interval(Enable)"=FALSE, "State Machine"=w462, "State_Machine_Class in"=w460) -> ()  [unwired: 7 in, 2 out]
          }
        }
      }
      event "UnLoad_Panel": Value Change {
        # "Do not using Shift Register to ignore some case Error"
        # "Not require\nUsing -> Auto Dispose Ref(True)"
        n205 = event-data() -> ()  [unwired: 1 in, 1 out]
        n206 = for {
          tunnel: w473 -> [w478] mode=indexing
          tunnel: w469 -> [w475]
          tunnel: [w474] -> w468
          i -> [w477]
          n207 = case shown="0, Default" w477 {
            tunnel: w475 -> [w487 w490 w492 w494 w496 w498 w500 w502 w504 w506]
            tunnel: w478 -> [_ _ _ _ _ _ _ _ _ _]
            tunnel: [w488 w489 w491 w493 w495 w497 w499 w501 w503 w505] -> w476
            frame 0, Default {
              n208 = invoke on="Panel 1" class="SubPnl" method="Remove VI"(error in=w487) -> (error out=w488:errorcluster)  [unwired: 2 in, 2 out]
            }
            frame 1 {
              n209 = invoke on="Panel 2" class="SubPnl" method="Remove VI"(error in=w490) -> (error out=w489:errorcluster)  [unwired: 2 in, 2 out]
            }
            frame 2 {
              n210 = invoke on="Panel 3" class="SubPnl" method="Remove VI"(error in=w492) -> (error out=w491:errorcluster)  [unwired: 2 in, 2 out]
            }
            frame 3 {
              n211 = invoke on="Panel 4" class="SubPnl" method="Remove VI"(error in=w494) -> (error out=w493:errorcluster)  [unwired: 2 in, 2 out]
            }
            frame 4 {
              n212 = invoke on="Panel 5" class="SubPnl" method="Remove VI"(error in=w496) -> (error out=w495:errorcluster)  [unwired: 2 in, 2 out]
            }
            frame 5 {
              n213 = invoke on="Panel 6" class="SubPnl" method="Remove VI"(error in=w498) -> (error out=w497:errorcluster)  [unwired: 2 in, 2 out]
            }
            frame 6 {
              n214 = invoke on="Panel 7" class="SubPnl" method="Remove VI"(error in=w500) -> (error out=w499:errorcluster)  [unwired: 2 in, 2 out]
            }
            frame 7 {
              n215 = invoke on="Panel 8" class="SubPnl" method="Remove VI"(error in=w502) -> (error out=w501:errorcluster)  [unwired: 2 in, 2 out]
            }
            frame 8 {
              n216 = invoke on="Panel 9" class="SubPnl" method="Remove VI"(error in=w504) -> (error out=w503:errorcluster)  [unwired: 2 in, 2 out]
            }
            frame 9 {
              n217 = invoke on="Panel 10" class="SubPnl" method="Remove VI"(error in=w506) -> (error out=w505:errorcluster)  [unwired: 2 in, 2 out]
            }
          }
          n218 = disable-structure shown="Enabled" {
            disable-tunnel: [w484 w486] -> w480
            disable-tunnel: [w483 w485] -> w479
            disable-tunnel: w478 -> [w482 w486]
            disable-tunnel: w476 -> [w481 w485]
            frame Disabled {
              n219 = invoke class="VI" method="Abort VI"(reference=w482, error in=w481) -> (reference out=w484:refnum<vi>, error out=w483:errorcluster)  [unwired: 1 in, 1 out]
            }
            frame Enabled {
            }
          }
          n220 = Close Reference(reference=w480, error in (no error)=w479) -> (error out=w474:errorcluster)
        }
        n221 = property on="UnLoad_Panel" class="Bool"(error in=w468, "DisabledEnum"=T1."Disabled and Grayed Out" ("Disabled")) -> (error out=w470:errorcluster)  [unwired: 1 in, 1 out]
        n222 = property on="Load_Panel" class="Bool"(error in=w470, "DisabledEnum"=T1."Enabled" ("Disabled")) -> (error out=w465:errorcluster)  [unwired: 1 in, 1 out]
        n223 = property on="Panel List" class="LstBox (strict)"(error in=w465, "Item Names"=string[] []) -> ()  [unwired: 1 in, 2 out]
      }
      event "Stop": Value Change {
        n224 = event-data() -> ()  [unwired: 1 in, 1 out]
        n225 = Two Button Dialog(message="Exit Confirm !") -> (T button?=w509:bool)  [unwired: 2 in]
        n226 = local write "Stop"(w509) -> ()
      }
    }
  }
  n227 = while {
    i -> [w512]
    stop <- w513 stop-if-true
    # "This is Simulate Interrupting Parallel Call Lock State at the Same Action of Own vi on Subpanel\n** It's Take Time when resume atfer Unlock"
    n228 = disable-structure shown="Disabled" {
      disable-tunnel: w512 -> [w516 _]
      frame Disabled {
        n229 = local read "HSMO[]"() -> (w520:refnum<class "Hyper_State_Machine.lvclass">[])
        n230 = Equal To 0?(x=w516) -> (x = 0?=w517:bool)
        n231 = call "Elapsed Time"("Reset"=w517) -> ("Time has Elapsed"=w515:bool)  [unwired: 11 in, 7 out]
        n232 = Empty Array?(array=w520) -> (empty?=w518:bool)
        n233 = And(x=w518, y=w515) -> (x .and. y?=w519:bool)
        n234 = case shown="False" w519 {
          tunnel: w520 -> [w521 _]
          frame False {
            n235 = for {
              tunnel: T3 {"Action_Mode (Get)"=enum."Get", "Action_Set (False)"=FALSE, "State_In (Wait)"="Lock"} ("Parameter") -> [w529]
              tunnel: w521 -> [w528] mode=indexing
              shift-right: [w526] -> _
              shift-left: errorcluster {"status"=FALSE, "code"=0, "source"=""} ("error out") -> [w527]
              tunnel: [w525] -> w524 mode=indexing
              n236 = call-dynamic "State_Lock_Unlock.vi"("error in (no error)"=w527, "Parameter"=w529, "State_Machine_Class in"=w528) -> ("error out"=w526:errorcluster, "Action_Get"=w530:bool)  [unwired: 6 in, 1 out]
              n237 = Boolean To (0,1)(Boolean=w530) -> (0, 1=w525:i16)
            }
            "Lock Status" <- w524
          }
          frame True {
          }
        }
      }
      frame Enabled {
      }
    }
    n238 = local read "System_Delay(s)"() -> (w514:dbl)
    n239 = local read "Stop"() -> (w513:bool)
    n240 = call <vilib>:"High Resolution Polling Wait.vi"("seconds to wait"=w514) -> ()  [unwired: 10 in, 1 out]
  }
  n241 = for {
    tunnel: w29 -> [w537] mode=indexing
    shift-right: [w534] -> w25
    shift-left: w28 -> [w533]
    i -> [w532]
    n242 = case shown="1" w532 {
      tunnel: w533 -> [w544 w547 w549 w551 w553 w555 w557 w559 w561 w563]
      tunnel: [w545 w546 w548 w550 w552 w554 w556 w558 w560 w562] -> w531
      frame 0, Default {
        n243 = invoke on="Panel 1" class="SubPnl" method="Remove VI"(error in=w544) -> (error out=w545:errorcluster)  [unwired: 2 in, 2 out]
      }
      frame 1 {
        n244 = invoke on="Panel 2" class="SubPnl" method="Remove VI"(error in=w547) -> (error out=w546:errorcluster)  [unwired: 2 in, 2 out]
      }
      frame 2 {
        n245 = invoke on="Panel 3" class="SubPnl" method="Remove VI"(error in=w549) -> (error out=w548:errorcluster)  [unwired: 2 in, 2 out]
      }
      frame 3 {
        n246 = invoke on="Panel 4" class="SubPnl" method="Remove VI"(error in=w551) -> (error out=w550:errorcluster)  [unwired: 2 in, 2 out]
      }
      frame 4 {
        n247 = invoke on="Panel 5" class="SubPnl" method="Remove VI"(error in=w553) -> (error out=w552:errorcluster)  [unwired: 2 in, 2 out]
      }
      frame 5 {
        n248 = invoke on="Panel 6" class="SubPnl" method="Remove VI"(error in=w555) -> (error out=w554:errorcluster)  [unwired: 2 in, 2 out]
      }
      frame 6 {
        n249 = invoke on="Panel 7" class="SubPnl" method="Remove VI"(error in=w557) -> (error out=w556:errorcluster)  [unwired: 2 in, 2 out]
      }
      frame 7 {
        n250 = invoke on="Panel 8" class="SubPnl" method="Remove VI"(error in=w559) -> (error out=w558:errorcluster)  [unwired: 2 in, 2 out]
      }
      frame 8 {
        n251 = invoke on="Panel 9" class="SubPnl" method="Remove VI"(error in=w561) -> (error out=w560:errorcluster)  [unwired: 2 in, 2 out]
      }
      frame 9 {
        n252 = invoke on="Panel 10" class="SubPnl" method="Remove VI"(error in=w563) -> (error out=w562:errorcluster)  [unwired: 2 in, 2 out]
      }
    }
    n253 = disable-structure shown="Disabled" {
      disable-tunnel: w537 -> [w541 w543]
      disable-tunnel: [w540 w543] -> w536
      disable-tunnel: [w539 w542] -> w535
      disable-tunnel: w531 -> [w538 w542]
      frame Disabled {
        n254 = invoke class="VI" method="Abort VI"(reference=w541, error in=w538) -> (reference out=w540:refnum<vi>, error out=w539:errorcluster)  [unwired: 1 in, 1 out]
      }
      frame Enabled {
      }
    }
    n255 = Close Reference(reference=w536, error in (no error)=w535) -> (error out=w534:errorcluster)
  }
  n256 = for {
    tunnel: w10 -> [w566] mode=indexing
    shift-right: [w565] -> w8
    shift-left: errorcluster {"status"=FALSE, "code"=0, "source"=""} ("error out") -> [w564]
    n257 = call-dynamic "State_Destroy.vi"("error in (no error)"=w564, "State_Machine_Class in"=w566) -> ("error out"=w565:errorcluster)  [unwired: 9 in]
  }
  n258 = call <vilib>:"Simple Error Handler.vi"("error in (no error)"=w8) -> ()  [unwired: 4 in, 5 out]
  n259 = invoke class="VI" method="FP.Close"(error in=w25) -> (error out=w26:errorcluster)  [unwired: 2 in, 2 out]
  n260 = call <vilib>:"Simple Error Handler.vi"("error in (no error)"=w26) -> ("error out"=w24:errorcluster)  [unwired: 4 in, 4 out]
  n261 = disable-structure shown="RUN_TIME_ENGINE==True" {
    disable-tunnel: w24 -> [_ _]
    frame condition #0 {
      n262 = Quit LabVIEW() -> ()  [unwired: 1 in]
    }
    frame condition #1 (active) {
    }
  }
